vi "Get PathArray.vi"(8 "error in (no error)":errorcluster, 11 "PathArrayMsg in":refnum<class "PathArrayMsg.lvclass">) -> (0 "error out":errorcluster, 2 "Message Data":path[](array[path]), 3 "PathArrayMsg out":refnum<class "PathArrayMsg.lvclass">)   [LabVIEW 2013, in "LapDog.Messaging.v3.NativeArrays.lvlib" / "PathArrayMsg.lvclass"]
doc: "Returns the data contained in the message.\n\nThis method executes regardless of the error in state."
uses:
  PathArrayMsg.lvclass
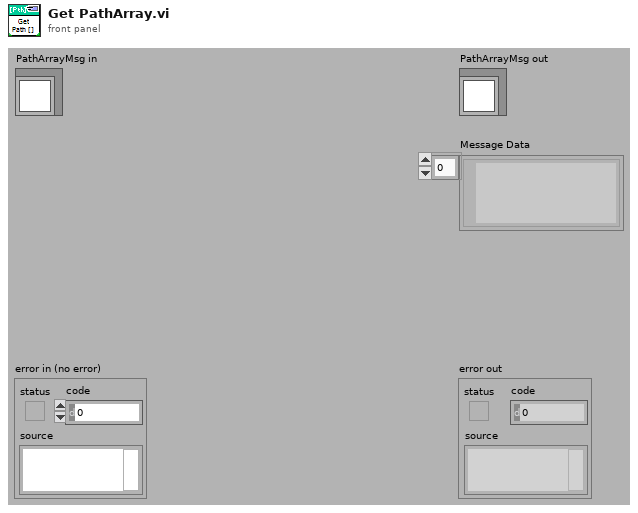
[diagram p1: front panel]
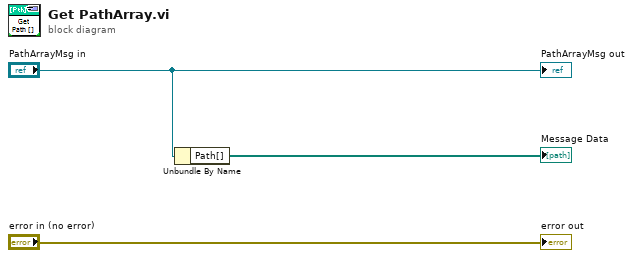
[diagram p0: block diagram]
diagram:
  n1 = Unbundle By Name("PathArrayMsg in") -> ("Path[]"=→"Message Data":path[])
  "error out" <- "error in (no error)"
  "PathArrayMsg out" <- "PathArrayMsg in"
